vi "Execute Value Update Policy.vi"(8 "error in (no error)":errorcluster, 9 "Publish Time":timestamp, 10 "New Topic Value":variant, 11 "WriteWhenVisibleSubscription In":refnum<class "WriteWhenVisibleSubscription.lvclass">) -> (0 "error out":errorcluster, 3 "WriteWhenVisibleSubscription Out":refnum<class "WriteWhenVisibleSubscription.lvclass">)   [LabVIEW 2017, in "SubscriptionPolicy.lvlib" / "WriteWhenVisibleSubscription.lvclass"]
uses:
  WriteWhenVisibleSubscription.lvclass
  C:/Git/mva-framework/Source/Framework/IMediator/ISubscriptionPolicy/ISubscriptionPolicy.lvclass
  WriteWhenVisibleSubscription.lvclass/WriteWhenVisibleSubscription.ctl
  IMediator/ISubscriptionPolicy/ISubscriptionPolicy.lvclass/ISubscriptionPolicy.ctl
  gpm_packages/@cs/transport/Source/ITransport/Transport Data.vi
  gpm_packages/@cs/transport/Source/ITransport/ITransport.lvclass
  IMediator/ISubscriptionPolicy/ISubscriptionPolicy.lvclass
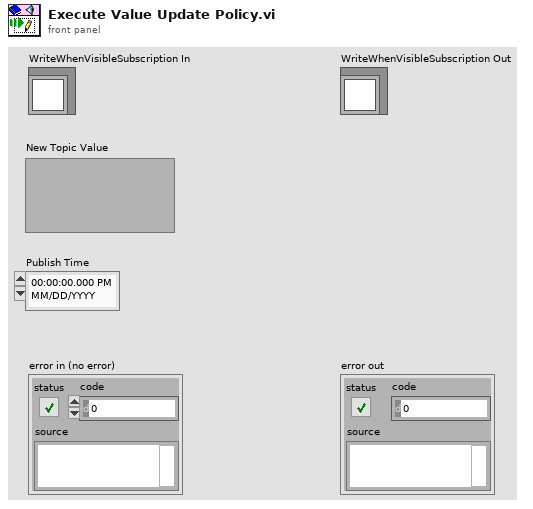
[diagram p1: front panel]
types:
  T1 = enum32{"Invalid", "Standard", "Closed", "Hidden", "Minimized", "Maximized"}
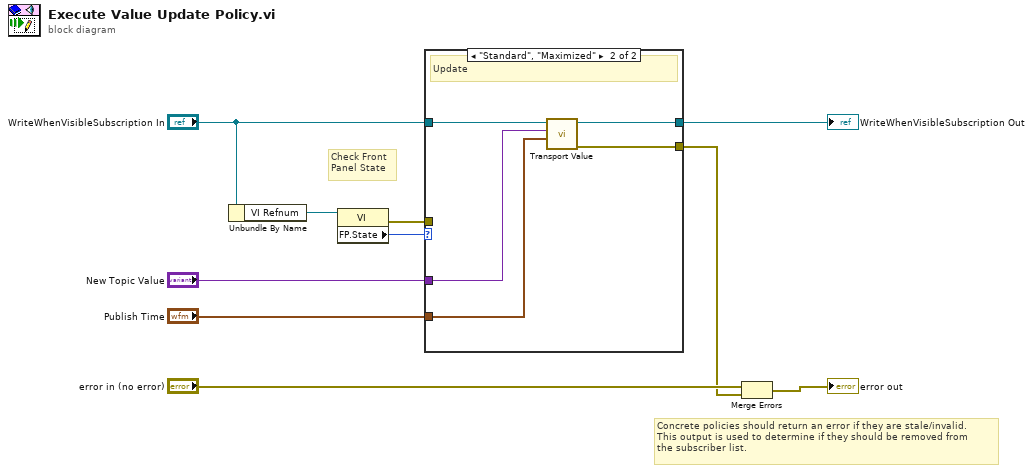
[diagram p0: block diagram]
diagram:
  # "Check Front\nPanel State"
  # "Concrete policies should return an error if they are stale/invalid.\nThis output is used to determine if they should be removed from\nthe subscriber list."
  n1 = Unbundle By Name("WriteWhenVisibleSubscription In") -> ("VI Refnum"=w3:refnum<vi>)
  n2 = property class="VI"(reference=w3) -> (error out=w7:errorcluster, "FP.State"=w8:T1)  [unwired: 1 in, 1 out]
  n3 = case shown="\"Standard\", \"Maximized\"" w8 {
    tunnel: "New Topic Value" -> [_ w14]
    tunnel: "Publish Time" -> [_ w13]
    tunnel: [w12 w15] -> w4
    tunnel: w7 -> [w12 _]
    tunnel: "WriteWhenVisibleSubscription In" -> [w11 w17]
    tunnel: [w11 w16] -> w1
    frame Default {
      # "No update"
    }
    frame "Standard", "Maximized" {
      # "Update"
      n4 = call "Transport Value.vi"("Publish Time"=w13, "Value"=w14, "ISubscriptionPolicy in"=w17) -> ("error out"=w15:errorcluster, "ISubscriptionPolicy out"=w16:refnum<class "WriteWhenVisibleSubscription.lvclass">)  [unwired: 7 in]
    }
  }
  "WriteWhenVisibleSubscription Out" <- w1
  n5 = Merge Errors("error in (no error)", w4) -> (→"error out":errorcluster)
